vi "Step Delete.vi"(0 "VISA resource name":refnum<visa-resource-name>, 7 "Step Number (0 = Active Step)":i32 min=0 max=60, 11 "error in (no error)":errorcluster) -> (4 "VISA resource name out":refnum<visa-resource-name>, 15 "error out":errorcluster)   [LabVIEW 2020, in "Associated Research 78XX Series.lvlib"]
doc: "SD <step number>\nDeletes the step indicated by the number from the setup file sequence. All step after this\nstep will move up and be renumbered accordingly."
uses:
  <instrlib>/Associated Research 78XX Series/Associated Research 78XX Series.lvlib
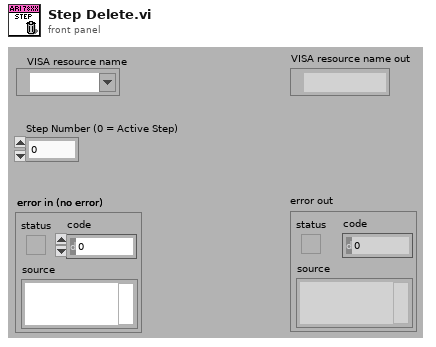
[diagram p1: front panel]
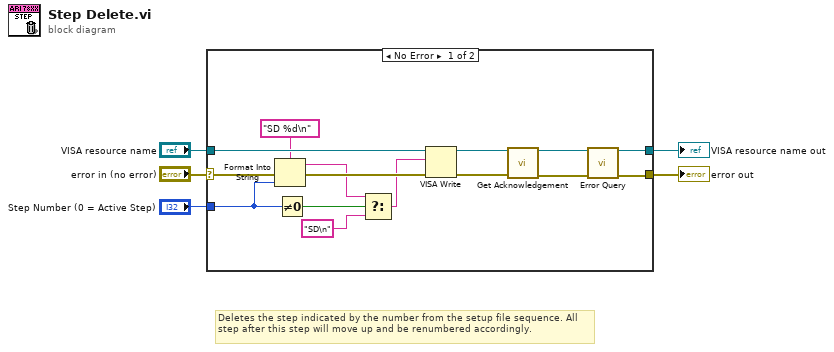
[diagram p0: block diagram]
diagram:
  # "Deletes the step indicated by the number from the setup file sequence. All step after this step will move up and be renumbered accordingly."
  n1 = case shown="No Error" "error in (no error)" {
    selector: "error in (no error)" -> [w17 w22]
    tunnel: [w15 w22] -> w4
    tunnel: [w19 w21] -> w2
    tunnel: "VISA resource name" -> [w20 w21]
    tunnel: "Step Number (0 = Active Step)" -> [w12 _]
    frame No Error {
      n2 = Format Into String(format string="SD %d\n" ("\"False\" Command"), error in=w17, w12) -> (resulting string=w10:string, error out=w16:errorcluster)  [unwired: 1 in]
      n3 = Not Equal To 0?(x=w12) -> (x != 0?=w13:bool)
      n4 = Select(t=w10, s=w13, f="SD\n") -> (s? t:f=w11:string)
      n5 = VISA Write(VISA resource name=w20, write buffer=w11, error in (no error)=w16) -> (VISA resource name out=w7:refnum<visa-resource-name>, error out=w6:errorcluster)  [unwired: 1 out]
      n6 = call <instrlib>:"Get Acknowledgement.vi"("VISA resource name"=w7, "error in (no error)"=w6) -> ("VISA resource name out"=w9:refnum<visa-resource-name>, "error out"=w8:errorcluster)  [unwired: 12 in]
      n7 = call <instrlib>:"Error Query.vi"("VISA resource name"=w9, "error in (no error)"=w8) -> ("VISA resource name out"=w19:refnum<visa-resource-name>, "error out"=w15:errorcluster)  [unwired: 10 in, 2 out]
    }
    frame Error {
    }
  }
  "error out" <- w4
  "VISA resource name out" <- w2
